vi "Process.vi"(8 "error in":errorcluster, 11 "MauiTemplate":refnum<class "MauiTemplate.lvclass">) -> (0 "error out":errorcluster, 3 "MauiTemplate out":refnum<class "MauiTemplate.lvclass">)   [LabVIEW 2016, in "MauiTemplate.lvclass"]
doc: "---------------------------------------------------------------\nJKI State Machine Objects™\nhttp://jki.net/state-machine-objects/\nCopyright (C) 2005-2015, JKI <info@jki.net>\nALL RIGHTS RESERVED"
uses:
  MauiTemplate.lvclass
  C:/Program Files (x86)/National Instruments/LabVIEW 2016/vi.lib/JKI/JKI SMO/SMO/SMO.lvclass
  C:/Program Files (x86)/National Instruments/LabVIEW 2016/vi.lib/Levylab/MAUI/MAUI.lvclass
  C:/Program Files (x86)/National Instruments/LabVIEW 2016/vi.lib/JKI/JKI SMO/SMO.UI/SMO.UI.lvclass
  <vilib>/JKI/JKI SMO/SMO/Typedefs/Parent Call--Enum.ctl
  <vilib>/Levylab/MAUI/Typedefs/PanelData.ctl
  <vilib>/Levylab/MAUI/MAUI.lvclass
  <vilib>/JKI/JKI SMO/SMO/SMO.lvclass
  <vilib>/JKI/JKI SMO/SMO.UI/SMO.UI.lvclass
panel:
  out "Title":string
  in  "Right Ring":u16(ring)
  in  "Left Ring":u16(ring)
  # "For instructions on how to use the JKI State Machine Objects, examples and video tutorials, visit:\nhttp://jki.net/state-machine-objects/\n\nJKI State Machine Objects™\nhttp://jki.net/state-machine-objects/\nCopyright (C) 2005-2015, JKI <info@jki.net>\nALL RIGHTS RESERVED"
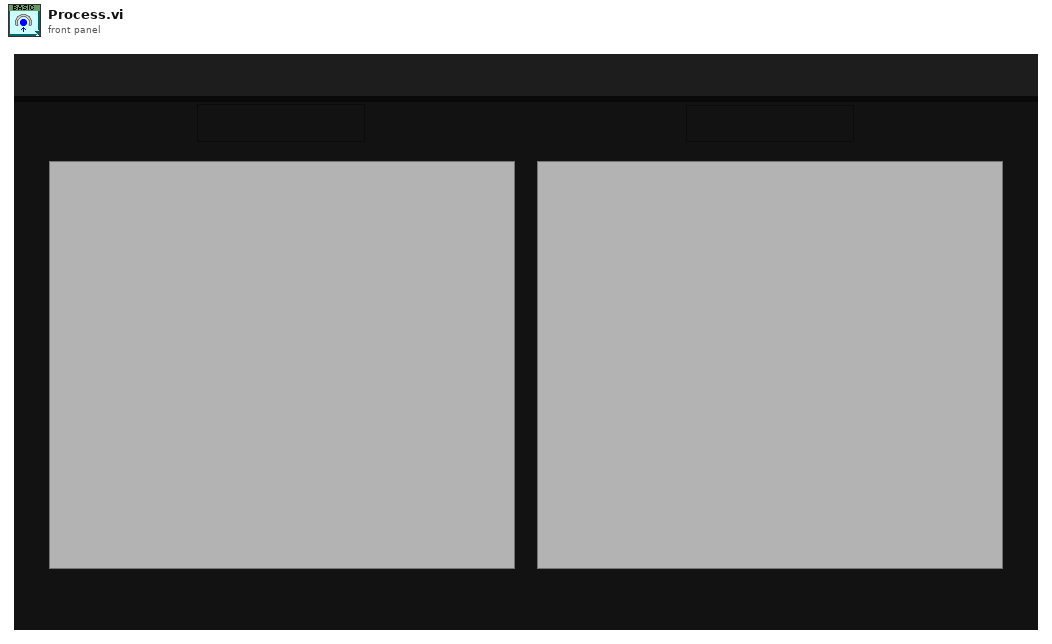
[diagram p1: front panel]
types:
  T1 = typedef "SMO.lvclass/Parent Call--Enum.ctl" = enum16{"Allows parent to run", "Does not request parent to run"}
  T2 = enum32{"invalid app kind", "Development System", "Run Time System", "Student Edition", "Embedded LabVIEW", "Evaluation", "Custom"}
  T3 = enum32{"Invalid", "Standard", "Closed", "Hidden", "Minimized", "Maximized"}
  T4 = enum32{"Bad", "Idle", "Run top level", "Running"}
  T5 = typedef "MAUI.lvclass/PanelData.ctl" = cluster{"Subpanel":refnum<vi>, "Ring":refnum<vi>, "Active":i32}
  T6 = cluster{"Core":cluster{"Current VI Reference":refnum<vi>, "Close Panel on Exit?":bool, "error":errorcluster}, "Self Reference":refnum<class "MauiTemplate.lvclass">, "Your string data":string, "Active Left":i32, "Active Right":i32}
  T7 = cluster{"Current VI Reference":refnum<vi>, "Close Panel on Exit?":bool, "error":errorcluster}
  T8 = typedef "SMO.lvclass/Protected Events.ctl" = cluster{"StopProcesses":refnum<user-event>, "AbortProcesses":refnum<user-event>, "Config Changed":refnum<user-event>, "Dependency":refnum<user-event>}
  T9 = typedef "MAUI.lvclass/PublicEvents--Cluster.ctl" = cluster{"ReadyForInfo ":refnum<user-event>}
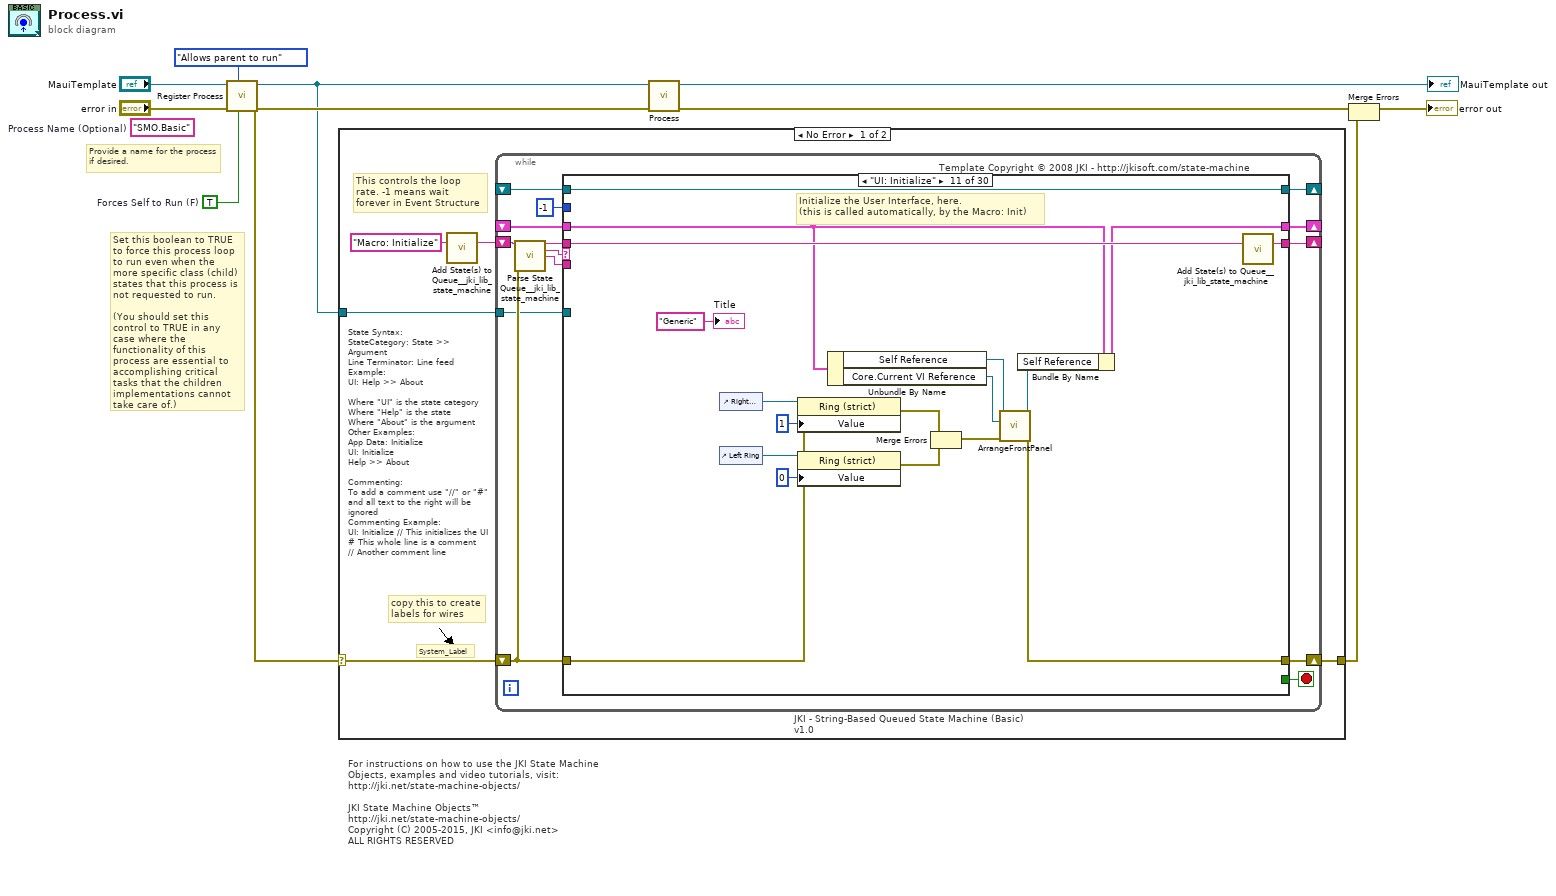
[diagram p0: block diagram]
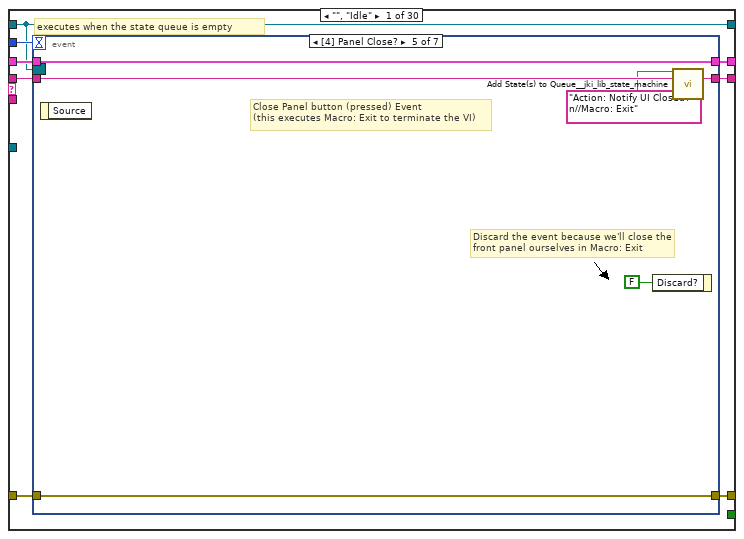
[diagram p2: hidden frame]
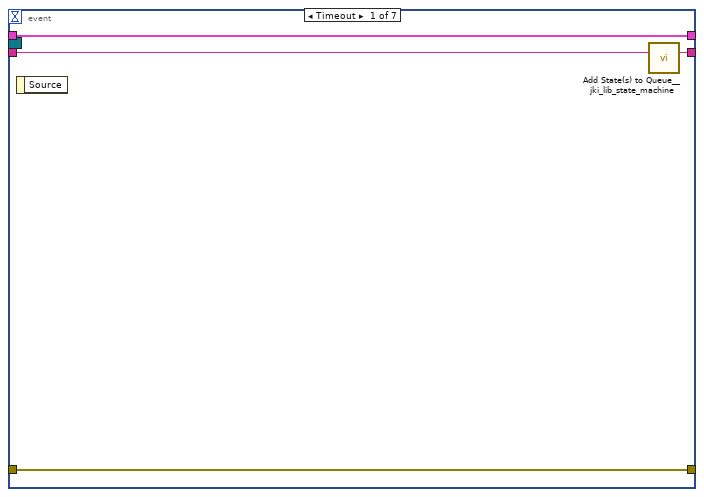
[diagram p3: hidden frame]
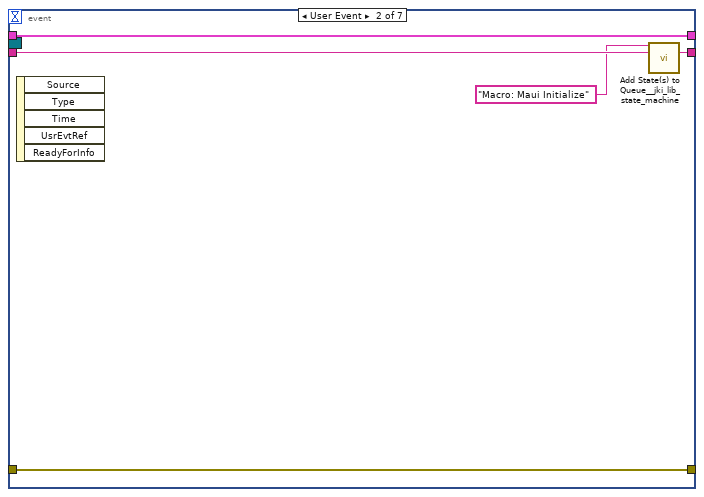
[diagram p4: hidden frame]
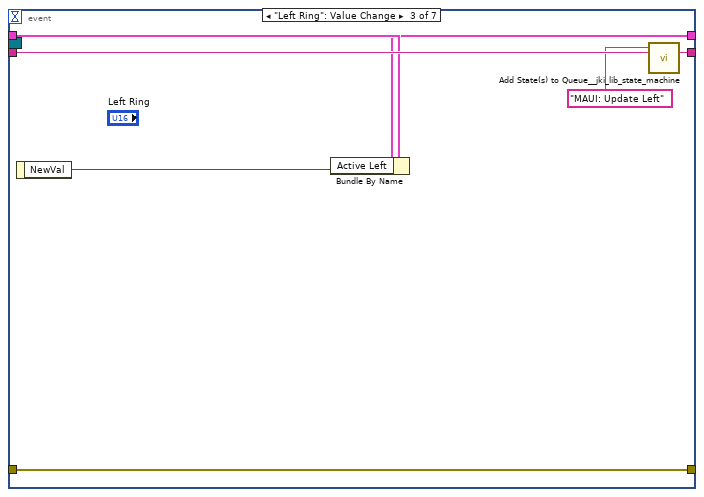
[diagram p5: hidden frame]
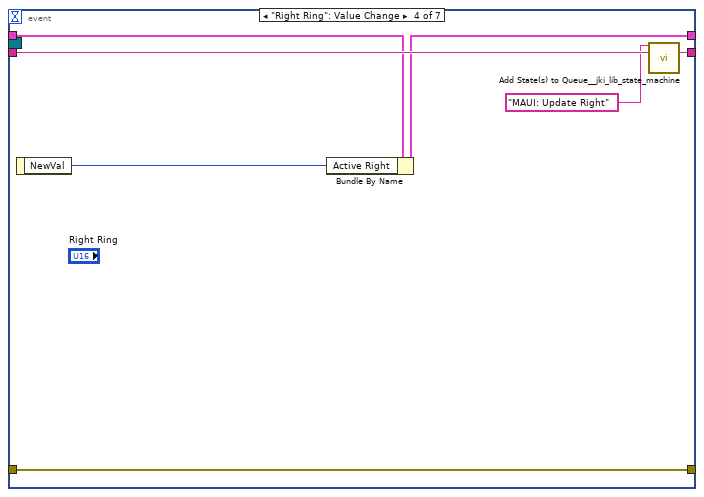
[diagram p6: hidden frame]
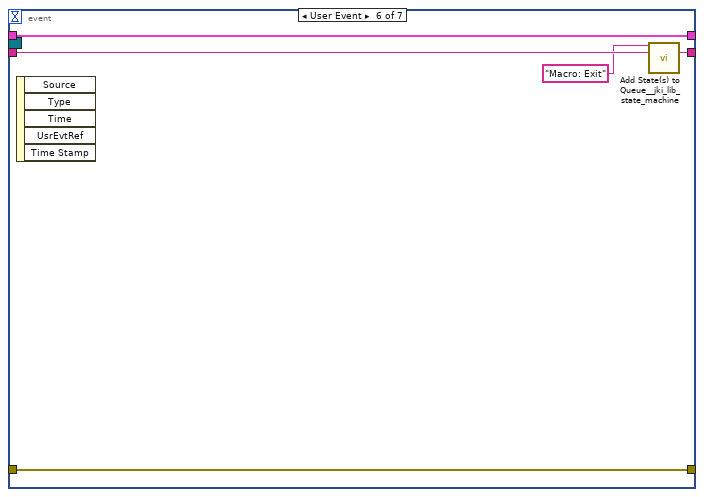
[diagram p7: hidden frame]
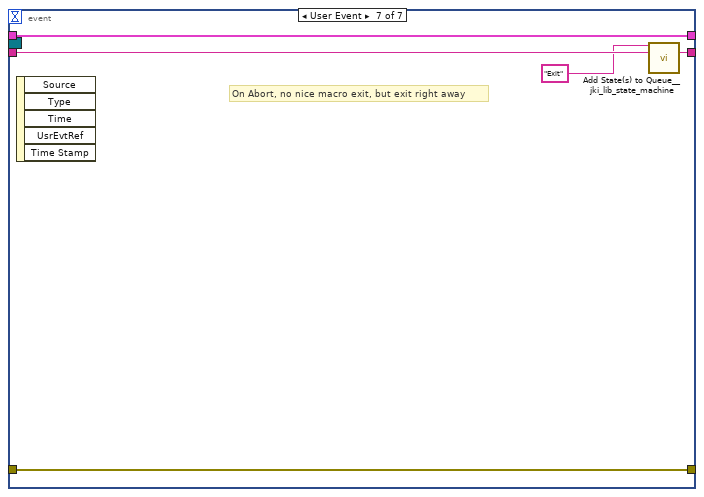
[diagram p8: hidden frame]
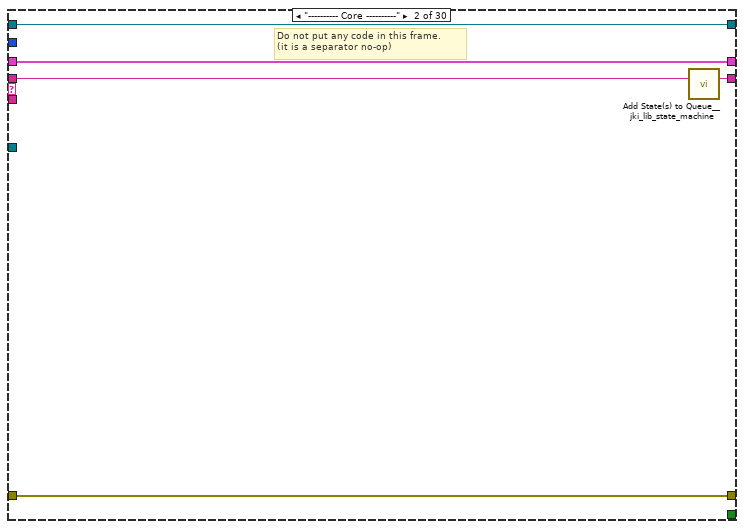
[diagram p9: hidden frame]
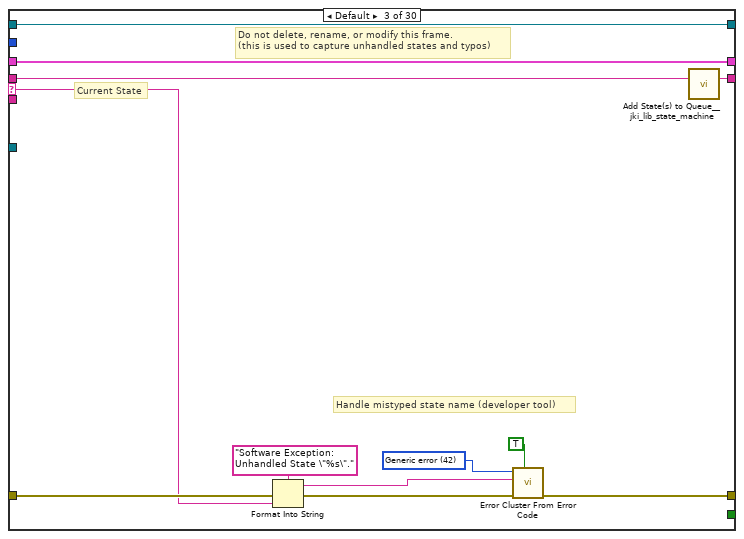
[diagram p10: hidden frame]
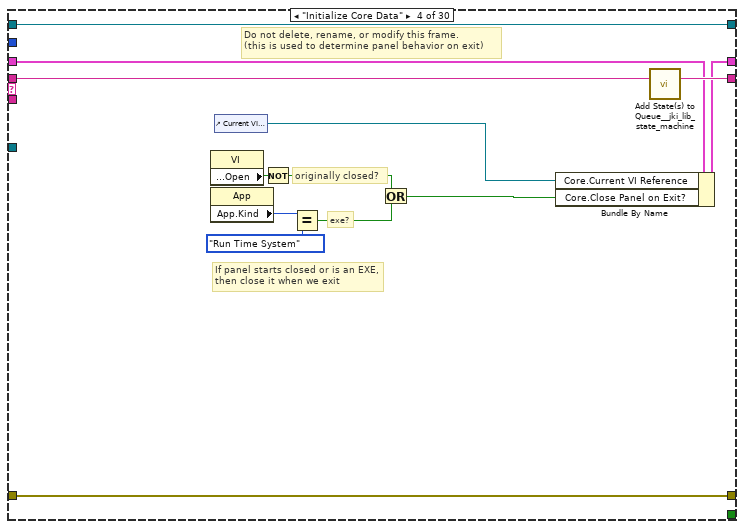
[diagram p11: hidden frame]
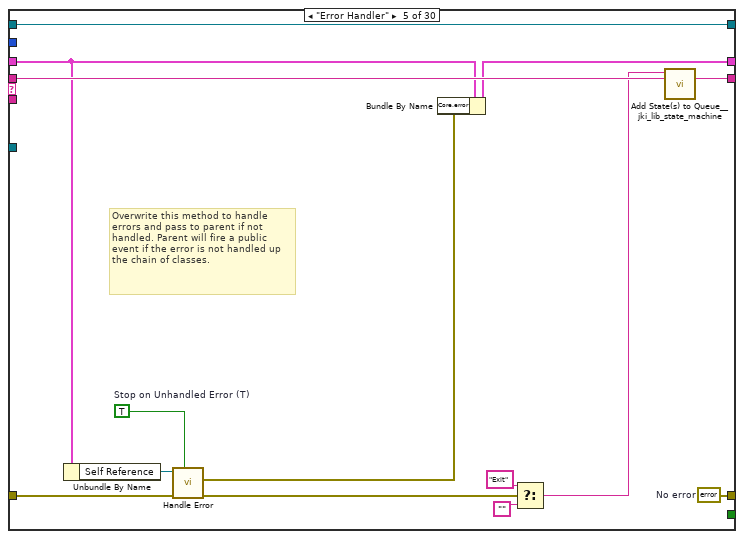
[diagram p12: hidden frame]
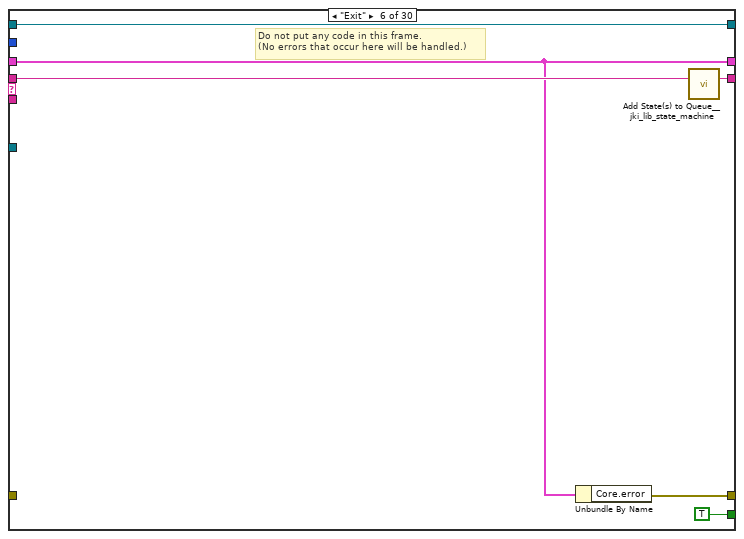
[diagram p13: hidden frame]
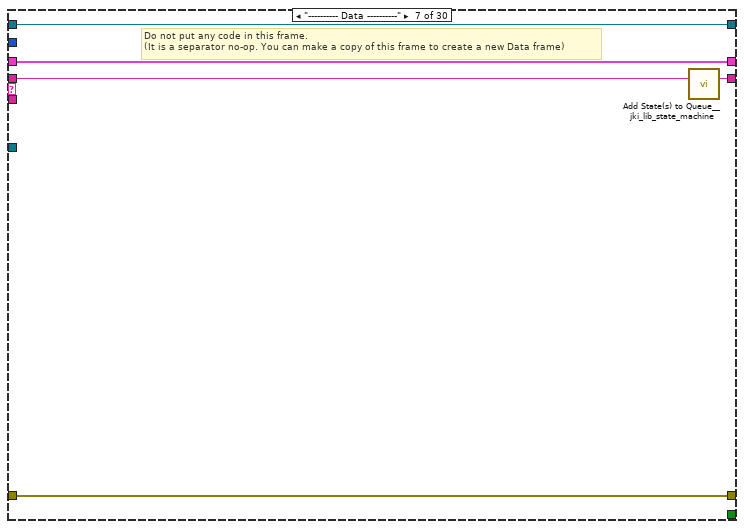
[diagram p14: hidden frame]
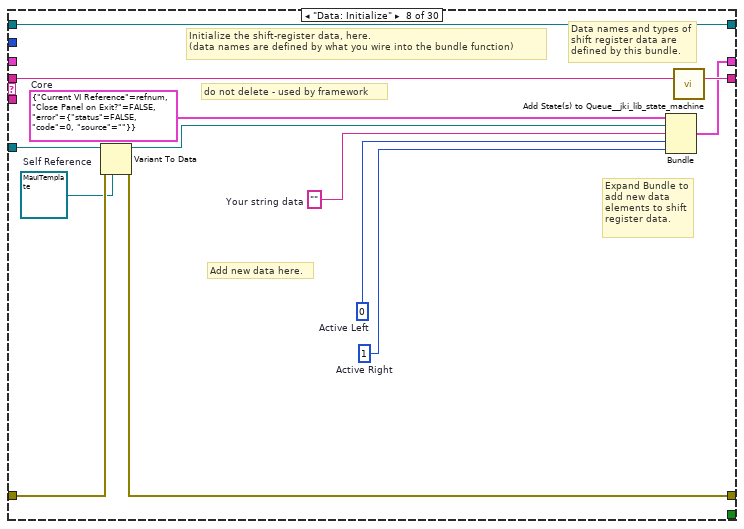
[diagram p15: hidden frame]
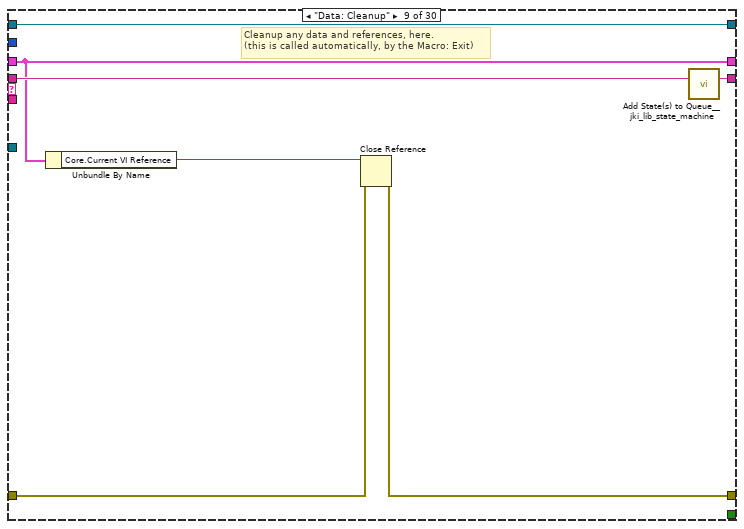
[diagram p16: hidden frame]
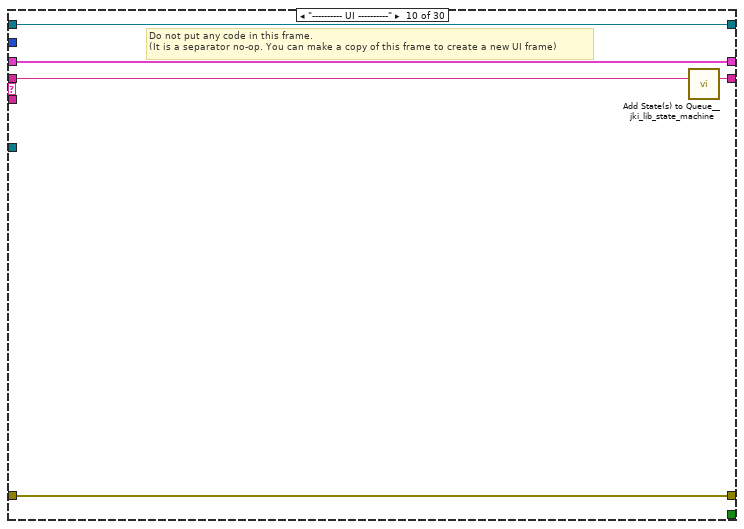
[diagram p17: hidden frame]
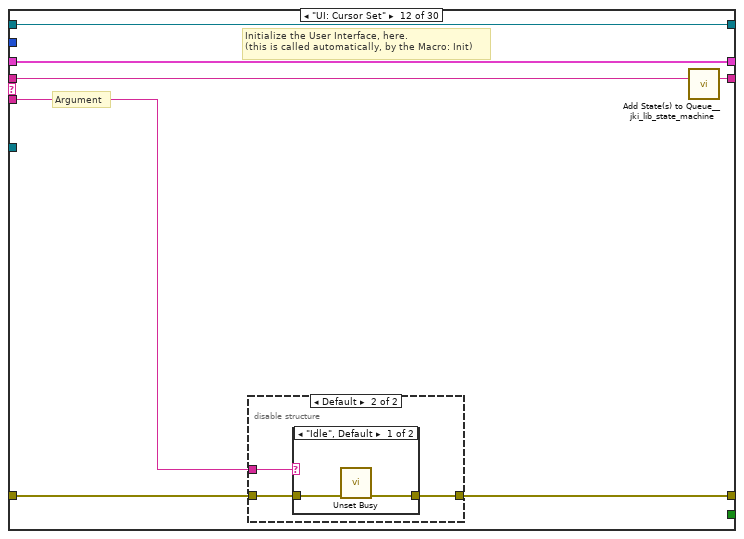
[diagram p18: hidden frame]
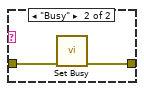
[diagram p20: hidden frame]
diagram:
  w2 = TRUE  # Forces Self to Run (F)
  (unwired) "SMO.Basic"  # Process Name (Optional)
  # "Provide a name for the process\nif desired."
  # "Set this boolean to TRUE to force this process loop to run even when the more specific class (child) states that this process is not requested to run.\n\n(You should set this control to TRUE in any case where the functionality of this process are essential to accomplishing critical tasks that the children implementations cannot take care of.)"
  # "For instructions on how to use the JKI State Machine Objects, examples and video tutorials, visit:\nhttp://jki.net/state-machine-objects/\n\nJKI State Machine Objects™\nhttp://jki.net/state-machine-objects/\nCopyright (C) 2005-2015, JKI <info@jki.net>\nALL RIGHTS RESERVED"
  n1 = call <vilib>:"Register Process.vi"("Forces Self to Run (F)"=w2, "Parent Call"=Parent_Call--Enum."Allows parent to run", "error in (no error)"="error in", "SMO"="MauiTemplate") -> ("error out"=w7:errorcluster, "SMO out"=w1:refnum<class "MauiTemplate.lvclass">)  [unwired: 6 in]
  n2 = case shown="No Error" w7 {
    selector: w7 -> [w12 w375]
    tunnel: w1 -> [w13 _]
    tunnel: [w11 w375] -> w4
    frame No Error {
      # "State Syntax:\nStateCategory: State >> Argument\nLine Terminator: Line feed\nExample:\nUI: Help >> About\n\nWhere \"UI\" is the state category\nWhere \"Help\" is the state\nWhere \"About\" is the argument\nOther Examples:\nApp Data: Initialize\nUI: Initialize\nHelp >> About\n\nCommenting:\nTo add a comment use \"//\" or \"#\" and all text to the right will be ignored\nCommenting Example:\nUI: Initialize // This initializes the UI\n# This whole line is a comment\n// Another comment line"
      # "copy this to create labels for wires"
      # "This controls the loop rate. -1 means wait forever in Event Structure"
      # "System_Label"
      n3 = call <vilib>:"Add State(s) to Queue__jki_lib_state_machine.vi"("State(s) in (\"\")"="Macro: Initialize") -> ("States Out"=w15:string)  [unwired: 14 in]
      n4 = while "JKI - String-Based Queued State Machine (Basic) v1.0" {
        shift-right: [w22] -> _
        shift-left: _ -> [w21]
        shift-right: [w25] -> w11
        shift-left: w12 -> [w19]
        shift-right: [w24] -> _
        shift-left: w15 -> [w26]
        tunnel: w13 -> [w18]
        shift-right: [w17] -> _
        shift-left: _ -> [w16]
        stop <- w23 stop-if-true
        # "Template Copyright © 2008 JKI - http://jkisoft.com/state-machine"
        n5 = call <vilib>:"Parse State Queue__jki_lib_state_machine.vi"("State Queue"=w26, "Error In (no error)"=w19) -> ("Remaining States"=w28:string, "Current State"=w29:string, "Arguments"=w27:string)  [unwired: 11 in]
        n6 = case shown="\"UI: Initialize\"" w29 {
          selector: w29 -> [_ _ w83 _ _ _ _ _ _ _ _ _ _ _ _ _ _ _ _ _ _ _ _ _ _ _ _ _ _ _]
          tunnel: w28 -> [w37 w81 w87 w106 w120 w126 w131 w144 w151 w156 w174 w181 w197 w229 w243 w249 w263 w268 w279 w284 w296 w302 w307 w314 w321 w326 w336 w346 w360 w374]
          tunnel: w27 -> [_ _ _ _ _ _ _ _ _ _ _ w175 w191 _ _ _ _ _ _ _ _ _ _ _ _ _ _ _ _ _]
          tunnel: w21 -> [w35 w78 w85 w97 w114 w122 w128 _ w146 w153 w168 w179 w193 w226 w239 w246 w254 w265 w276 w281 w294 w300 w305 w311 w317 w324 w333 w343 w352 w368]
          tunnel: [w34 w79 w89 w103 w115 w121 w129 w139 w147 w154 w164 w176 w194 w227 w241 w247 w261 w266 w270 w282 w290 w298 w303 w308 w318 w322 w328 w338 w354 w370] -> w25
          tunnel: w19 -> [w33 w79 w88 w103 w116 _ w129 w140 w148 w154 w160 w177 w195 w227 w241 w247 w261 w266 w271 w282 w291 w298 w303 w309 w318 w322 w327 w339 w355 w371]
          tunnel: [w36 w80 w86 w105 w119 w125 w130 w143 w150 w155 w173 w180 w196 w228 w242 w248 w262 w267 w278 w283 w295 w301 w306 w313 w320 w325 w335 w345 w359 w373] -> w24
          tunnel: [_ _ _ _ _ TRUE _ _ _ _ _ _ _ _ _ _ _ _ _ _ _ _ _ _ _ _ _ _ _ _] -> w23
          tunnel: [w32 w78 w85 w104 w113 w122 w128 w142 w146 w153 w167 w179 w193 w226 w239 w246 w254 w265 w276 w281 w294 w300 w305 w311 w316 w324 w332 w342 w351 w367] -> w22
          tunnel: -1 ("Timeout") -> [w31 _ _ _ _ _ _ _ _ _ _ _ _ _ _ _ _ _ _ _ _ _ _ _ _ _ _ _ _ _]
          tunnel: w18 -> [_ _ _ _ _ _ _ w137 _ _ _ _ _ _ _ _ _ _ _ _ _ _ _ _ _ _ _ _ _ _]
          tunnel: [w30 w77 w82 w94 w118 w123 w127 w135 w145 w152 w172 w178 w190 w225 w240 w245 w255 w264 w277 w280 w293 w299 w304 w312 w319 w323 w334 w344 w358 w372] -> w17
          tunnel: w16 -> [w30 w77 w82 w94 w118 w123 w127 w135 w145 w152 w172 w178 w190 w225 w240 w245 w255 w264 w277 w280 _ w299 w304 w312 w319 w323 w334 w344 w358 w372]
          frame "", "Idle" {
            # "executes when the state queue is empty"
            n7 = event shown="[4] Panel Close?" {
              selector: w30 -> [_ _ _ _ _ _ _]
              dyn-events: _ -> [_ _ _ _ _ _ _]
              timeout: w31 -> [_ _ _ _ _ _ _]
              tunnel: w37 -> [w41 w46 w53 w60 w66 w71 w76]
              tunnel: [w40 w45 w52 w59 w65 w70 w75] -> w36
              tunnel: w35 -> [w39 w44 w50 w57 w63 w68 w73]
              tunnel: [w38 w43 w51 w58 w64 w69 w74] -> w34
              tunnel: w33 -> [w38 w43 w51 w58 w64 w69 w74]
              tunnel: [w39 w44 w49 w56 w63 w68 w73] -> w32
              event Timeout {
                n8 = event-data() -> ()  [unwired: 1 in, 1 out]
                n9 = call <vilib>:"Add State(s) to Queue__jki_lib_state_machine.vi"("State(s) in (\"\")"=w41) -> ("States Out"=w40:string)  [unwired: 14 in]
              }
              event User Event {
                n10 = event-data() -> ()  [unwired: 1 in, 5 out]
                n11 = call <vilib>:"Add State(s) to Queue__jki_lib_state_machine.vi"("State(s) in Front (\"\")"="Macro: Maui Initialize", "State(s) in (\"\")"=w46) -> ("States Out"=w45:string)  [unwired: 13 in]
              }
              event "Left Ring": Value Change {
                n12 = event-data() -> ("NewVal"=w48:u16)  [unwired: 1 in]
                n13 = Bundle By Name(cluster=w50, "Active Left"=w48) -> (w49:T6)
                n14 = call <vilib>:"Add State(s) to Queue__jki_lib_state_machine.vi"("State(s) in Front (\"\")"="MAUI: Update Left", "State(s) in (\"\")"=w53) -> ("States Out"=w52:string)  [unwired: 13 in]
              }
              event "Right Ring": Value Change {
                n15 = event-data() -> ("NewVal"=w55:u16)  [unwired: 1 in]
                n16 = Bundle By Name(cluster=w57, "Active Right"=w55) -> (w56:T6)
                n17 = call <vilib>:"Add State(s) to Queue__jki_lib_state_machine.vi"("State(s) in Front (\"\")"="MAUI: Update Right", "State(s) in (\"\")"=w60) -> ("States Out"=w59:string)  [unwired: 13 in]
              }
              event Panel Close? {
                # "Discard the event because we'll close the front panel ourselves in Macro: Exit"
                # "Close Panel button (pressed) Event\n(this executes Macro: Exit to terminate the VI)"
                n18 = event-data() -> ()  [unwired: 1 in, 1 out]
                n19 = event-data("Discard?"=FALSE) -> ()  [unwired: 1 in, 1 out]
                n20 = call <vilib>:"Add State(s) to Queue__jki_lib_state_machine.vi"("State(s) in Front (\"\")"="Action: Notify UI Closed\n//Macro: Exit", "State(s) in (\"\")"=w66) -> ("States Out"=w65:string)  [unwired: 13 in]
              }
              event User Event {
                n21 = event-data() -> ()  [unwired: 1 in, 5 out]
                n22 = call <vilib>:"Add State(s) to Queue__jki_lib_state_machine.vi"("State(s) in Front (\"\")"="Macro: Exit", "State(s) in (\"\")"=w71) -> ("States Out"=w70:string)  [unwired: 13 in]
              }
              event User Event {
                # "On Abort, no nice macro exit, but exit right away"
                n23 = event-data() -> ()  [unwired: 1 in, 5 out]
                n24 = call <vilib>:"Add State(s) to Queue__jki_lib_state_machine.vi"("State(s) in Front (\"\")"="Exit", "State(s) in (\"\")"=w76) -> ("States Out"=w75:string)  [unwired: 13 in]
              }
            }
          }
          frame "---------- Core ----------" {
            # "Do not put any code in this frame.\n(it is a separator no-op)"
            n25 = call <vilib>:"Add State(s) to Queue__jki_lib_state_machine.vi"("State(s) in (\"\")"=w81) -> ("States Out"=w80:string)  [unwired: 14 in]
          }
          frame Default {
            w92 = 42 items=["No error", "Argument error", "Memory is full", "Out of zone", "End of file", "File already open", "Generic file I/O error", "File not found", "File permission error", "Disk is full", "Duplicate path", "Too many files open", "System feature not enabled", "Resource file not found", "Cannot add resource", "Resource not found", "Image not found", "Image memory error", "Pen does not exist", "Config type invalid", "Config token not found", "Config parse error", "Config memory error", "Bad external code format", "Bad external code offset", "External code not present", "Null window", "Destroy window error", "Null menu", "Print aborted", "Bad print record", "Print driver error", "Windows error during printing", "Memory error during printing", "Print dialog error", "Generic print error", "Invalid device refnum", "Device not found", "Device parameter error", "Device unit error", "Cannot open device", "Device call aborted", "Generic error", "Cancelled by user", "Object ID too low", "Object ID too high", "Object not in heap", "Unknown heap", "Unknown object (invalid DefProc)", "Unknown object (DefProc not in table)", "Message out of range", "Invalid (null) method", "Unknown message", "Manager call not supported", "Bad address", "Network operation in progress", "Network operation timed out", "Connection is busy", "Network attribute not supported", "Network error", "Address in use", "System out of memory", "Connection aborted", "Connection refused", "Not connected", "Already connected", "Connection closed", "Initialization error (interapplication manager)", "Bad occurrence", "Wait on unbound occurrence handler", "Occurrence queue overflow", "Datalog type conflict", "Unused", "Unrecognized type (interapplication manager)", "Memory corrupt", "Failed to make temporary DLL", "Old CIN version", "Drag socket not found", "Failed to load drop-object", "Failed to register OLE object", "Failed to release OLE object", "Format specifier type mismatch", "Unknown format specifier", "Too few format specifiers", "Too many format specifiers", "Scan failed", "Newer CIN version", "Error converting to variant", "Runtime menu error", "Password tampered", "Variant attribute not found", "Incompatible variant data type", "Event data is not available", "Event Store is not present", "Occurrence is not found", "Event Queue is not created", "Event info is not available", "Refnum passed is NULL", "Error retrieving Class GUID", "Error retrieving CoClass GUID", "Error retrieving TypeLib GUID.", "Bad built application magic bytes.", "Specific driver is different from the specific driver associated with the Logical Name.", "There is no session opened to the class driver.", "Max Error", "MAX - Error with config objects", "MAX - Error loading configuration", "MAX - Group not supported"]
            # "Current State"
            # "Do not delete, rename, or modify this frame.\n(this is used to capture unhandled states and typos)"
            # "Handle mistyped state name (developer tool)"
            n26 = Format Into String(format string="Software Exception: Unhandled State \"%s\"." ("message"), error in=w88, w83) -> (resulting string=w91:string, error out=w90:errorcluster)  [unwired: 1 in]
            n27 = call <vilib>:"Error Cluster From Error Code.vi"("show call chain? (False)"=TRUE, "error in (no error)"=w90, "error message (\"\")"=w91, "error code (0)"=w92) -> ("error out"=w89:errorcluster)  [unwired: 5 in]
            n28 = call <vilib>:"Add State(s) to Queue__jki_lib_state_machine.vi"("State(s) in (\"\")"=w87) -> ("States Out"=w86:string)  [unwired: 14 in]
          }
          frame "Initialize Core Data" {
            # "Do not delete, rename, or modify this frame.\n(this is used to determine panel behavior on exit)"
            # "originally closed?"
            # "exe?"
            # "If panel starts closed or is an EXE, then close it when we exit"
            n29 = property class="VI"() -> ("Front Panel.Open"=w102:bool)  [unwired: 2 in, 2 out]
            n30 = property class="App"() -> ("App.Kind"=w101:T2)  [unwired: 2 in, 2 out]
            n31 = control-ref of="Current VI Reference"() -> (w95:refnum<vi>)
            n32 = Not(x=w102) -> (.not. x?=w99:bool)
            n33 = Equal?(x=w101, y=T2."Run Time System" ("Application:Kind")) -> (x = y?=w98:bool)
            n34 = Or(x=w99, y=w98) -> (x .or. y?=w96:bool)
            n35 = Bundle By Name(cluster=w97, "Core.Current VI Reference"=w95, "Core.Close Panel on Exit?"=w96) -> (w104:T6)
            n36 = call <vilib>:"Add State(s) to Queue__jki_lib_state_machine.vi"("State(s) in (\"\")"=w106) -> ("States Out"=w105:string)  [unwired: 14 in]
          }
          frame "Error Handler" {
            w107 = TRUE  # Stop on Unhandled Error (T)
            w115 = errorcluster {"status"=FALSE, "code"=0, "source"=""}  # No error
            # "Overwrite this method to handle errors and pass to parent if not handled. Parent will fire a public event if the error is not handled up the chain of classes."
            n37 = Unbundle By Name(w114) -> ("Self Reference"=w117:refnum<class "MauiTemplate.lvclass">)
            n38 = call-dynamic "Handle Error.vi"("Stop on Unhandled Error (T)"=w107, "error in"=w116, "SMO"=w117) -> ("handling error"=w108:errorcluster, "Unhandled error"=w111:errorcluster)  [unwired: 6 in, 1 out]
            n39 = Bundle By Name(cluster=w114, "Core.error"=w111) -> (w113:T6)
            n40 = Select(t="Exit", s=w108, f="") -> (s? t:f=w112:string)
            n41 = call <vilib>:"Add State(s) to Queue__jki_lib_state_machine.vi"("State(s) in Front (\"\")"=w112, "State(s) in (\"\")"=w120) -> ("States Out"=w119:string)  [unwired: 13 in]
          }
          frame "Exit" {
            # "Do not put any code in this frame.\n(No errors that occur here will be handled.)"
            n42 = Unbundle By Name(w122) -> ("Core.error"=w121:errorcluster)
            n43 = call <vilib>:"Add State(s) to Queue__jki_lib_state_machine.vi"("State(s) in (\"\")"=w126) -> ("States Out"=w125:string)  [unwired: 14 in]
          }
          frame "---------- Data ----------" {
            # "Do not put any code in this frame.\n(It is a separator no-op. You can make a copy of this frame to create a new Data frame)"
            n44 = call <vilib>:"Add State(s) to Queue__jki_lib_state_machine.vi"("State(s) in (\"\")"=w131) -> ("States Out"=w130:string)  [unwired: 14 in]
          }
          frame "Data: Initialize" {
            w132 = 1  # Active Right
            w133 = 0  # Active Left
            w134 = T7 {"Current VI Reference"=refnum, "Close Panel on Exit?"=FALSE, "error"={"status"=FALSE, "code"=0, "source"=""}}  # Core
            w138 = refnum<class "MauiTemplate.lvclass"> refnum  # Self Reference
            w141 = ""  # Your string data
            # "do not delete - used by framework"
            # "Expand Bundle to add new data elements to shift register data."
            # "Add new data here."
            # "Data names and types of shift register data are defined by this bundle."
            # "Initialize the shift-register data, here.\n(data names are defined by what you wire into the bundle function)"
            n45 = Variant To Data(error in=w140, type=w138, Variant=w137) -> (data=w136:refnum<class "MauiTemplate.lvclass">, error out=w139:errorcluster)
            n46 = Bundle("Core"=w134, "Self Reference"=w136, "Your string data"=w141, "Active Left"=w133, "Active Right"=w132) -> (w142:T6)  [unwired: 1 in]
            n47 = call <vilib>:"Add State(s) to Queue__jki_lib_state_machine.vi"("State(s) in (\"\")"=w144) -> ("States Out"=w143:string)  [unwired: 14 in]
          }
          frame "Data: Cleanup" {
            # "Cleanup any data and references, here.\n(this is called automatically, by the Macro: Exit)"
            n48 = Unbundle By Name(w146) -> ("Core.Current VI Reference"=w149:refnum<vi>)
            n49 = Close Reference(reference=w149, error in (no error)=w148) -> (error out=w147:errorcluster)
            n50 = call <vilib>:"Add State(s) to Queue__jki_lib_state_machine.vi"("State(s) in (\"\")"=w151) -> ("States Out"=w150:string)  [unwired: 14 in]
          }
          frame "---------- UI ----------" {
            # "Do not put any code in this frame.\n(It is a separator no-op. You can make a copy of this frame to create a new UI frame)"
            n51 = call <vilib>:"Add State(s) to Queue__jki_lib_state_machine.vi"("State(s) in (\"\")"=w156) -> ("States Out"=w155:string)  [unwired: 14 in]
          }
          frame "UI: Initialize" {
            # "Initialize the User Interface, here.\n(this is called automatically, by the Macro: Init)"
            n52 = control-ref of="Right Ring"() -> (w171:refnum<vi>)
            n53 = control-ref of="Left Ring"() -> (w162:refnum<vi>)
            n54 = property class="Ring (strict)"(reference=w171, error in=w160, "Value"=u16 1) -> (error out=w157:errorcluster)  [unwired: 1 out]
            n55 = property class="Ring (strict)"(reference=w162, error in=w160, "Value"=u16 0) -> (error out=w158:errorcluster)  [unwired: 1 out]
            n56 = Unbundle By Name(w168) -> ("Self Reference"=w169:refnum<class "MauiTemplate.lvclass">, "Core.Current VI Reference"=w165:refnum<vi>)
            n57 = Merge Errors(w157, w158) -> (w159:errorcluster)
            n58 = call <vilib>:"ArrangeFrontPanel.vi"("error in (no error)"=w159, "This VI"=w165, "MAUI in"=w169) -> ("error out"=w164:errorcluster, "MAUI out"=w166:refnum<class "MauiTemplate.lvclass">)  [unwired: 7 in]
            n59 = Bundle By Name(cluster=w168, "Self Reference"=w166) -> (w167:T6)
            n60 = call <vilib>:"Add State(s) to Queue__jki_lib_state_machine.vi"("State(s) in (\"\")"=w174) -> ("States Out"=w173:string)  [unwired: 14 in]
            "Title" <- "Generic" ("Title")
          }
          frame "UI: Cursor Set" {
            # "Argument"
            # "Initialize the User Interface, here.\n(this is called automatically, by the Macro: Init)"
            n61 = disable-structure shown="Default" {
              disable-tunnel: w177 -> [w182 w185]
              disable-tunnel: [w182 w184] -> w176
              disable-tunnel: w175 -> [_ w183]
              frame condition #0 {
              }
              frame condition #1 (active) {
                n62 = case shown="\"Idle\", Default" w183 {
                  tunnel: w185 -> [w187 w189]
                  tunnel: [w186 w188] -> w184
                  frame "Idle", Default {
                    n63 = call <vilib>:"Unset Busy.vi"("error in (no error)"=w187) -> ("error out"=w186:errorcluster)  [unwired: 10 in]
                  }
                  frame "Busy" {
                    n64 = call <vilib>:"Set Busy.vi"("error in (no error)"=w189) -> ("error out"=w188:errorcluster)  [unwired: 9 in, 1 out]
                  }
                }
              }
            }
            n65 = call <vilib>:"Add State(s) to Queue__jki_lib_state_machine.vi"("State(s) in (\"\")"=w181) -> ("States Out"=w180:string)  [unwired: 14 in]
          }
          frame "UI: Front Panel State" {
            # "Argument"
            # "Set Front Panel Open or Closed\n(Usage: \"UI: Front Panel State >> Open|Close\")"
            n66 = Unbundle By Name(w193) -> ("Core.Current VI Reference"=w192:refnum<vi>)
            n67 = disable-structure shown="Default" {
              disable-tunnel: w195 -> [w201 w224]
              disable-tunnel: [w200 w224] -> w194
              disable-tunnel: w192 -> [w199 _]
              disable-tunnel: w191 -> [w198 _]
              frame condition #0 (active) {
                n68 = case shown="\"Close\"" w198 {
                  tunnel: w201 -> [w205 w218]
                  tunnel: [w207 w219] -> w200
                  tunnel: w199 -> [w206 w216]
                  frame "Open", Default {
                    n69 = property class="VI"(reference=w206, error in=w205) -> (reference out=w203:refnum<vi>, error out=w204:errorcluster, "FP.State"=w202:T3)
                    n70 = case shown="\"Closed\"" w202 {
                      tunnel: [w210 w213] -> w207
                      tunnel: w204 -> [w209 w213]
                      tunnel: w203 -> [w208 _]
                      frame "Closed" {
                        n71 = invoke class="VI" method="FP.Open"(reference=w208, error in=w209, "Activate"=TRUE, "State"=T3."Standard") -> (error out=w210:errorcluster)  [unwired: 1 in, 4 out]
                      }
                      frame Default {
                      }
                    }
                  }
                  frame "Close" {
                    n72 = property class="VI"(reference=w216, error in=w218) -> (reference out=w215:refnum<vi>, error out=w217:errorcluster, "FP.State"=w214:T3)
                    n73 = case shown="Default" w214 {
                      tunnel: [w220 w223] -> w219
                      tunnel: w217 -> [w220 w222]
                      tunnel: w215 -> [_ w221]
                      frame "Invalid", "Closed" {
                      }
                      frame Default {
                        n74 = invoke class="VI" method="FP.Close"(reference=w221, error in=w222) -> (error out=w223:errorcluster)  [unwired: 1 in, 2 out]
                      }
                    }
                  }
                }
              }
              frame condition #1 {
              }
            }
            n75 = call <vilib>:"Add State(s) to Queue__jki_lib_state_machine.vi"("State(s) in (\"\")"=w197) -> ("States Out"=w196:string)  [unwired: 14 in]
          }
          frame "---------- Macro ----------" {
            # "Do not put any code in this frame.\n(It is a separator no-op. You can make a copy of this frame to create a new Macro frame)"
            n76 = call <vilib>:"Add State(s) to Queue__jki_lib_state_machine.vi"("State(s) in (\"\")"=w229) -> ("States Out"=w228:string)  [unwired: 14 in]
          }
          frame "Macro: Initialize" {
            w234 = "UI: Initialize\nUI: Front Panel State >> Open"  # UI: Initialize UI: Front Panel State >> Open
            w230 = "Process: Sync"
            # "Initialization Macro\n(This is called once, when the VI starts)"
            n77 = control-ref of="This VI"() -> (w232:refnum<vi>)
            n78 = property class="VI"(reference=w232) -> ("Exec.State"=w231:T4)  [unwired: 1 in, 2 out]
            n79 = Equal?(x=w231, y=T4."Run top level") -> (x = y?=w237:bool)
            n80 = Select(t=w230, s=w237, f="") -> ()  [unwired: 1 out]
            n81 = call <vilib>:"Add State(s) to Queue__jki_lib_state_machine.vi"("State(s) in Front (\"\")"="Data: Initialize\nInitialize Core Data\nEvents: Register", "State(s) in (\"\")"=w230, "State(s) at Back (\"\")"=w234) -> ("States Out"=w233:string)  [unwired: 12 in]
            n82 = call <vilib>:"Add State(s) to Queue__jki_lib_state_machine.vi"("State(s) in Front (\"\")"=w233, "State(s) in (\"\")"=w243) -> ("States Out"=w242:string)  [unwired: 13 in]
          }
          frame "Macro: Maui Initialize" {
            # "Do not put any code in this frame.\n(It is a separator no-op. You can make a copy of this frame to create a new Macro frame)"
            n83 = call <vilib>:"Add State(s) to Queue__jki_lib_state_machine.vi"("State(s) in Front (\"\")"="MAUI: Send Left\nMAUI: Send Right\nMAUI: Update Left\nMAUI: Update Right", "State(s) in (\"\")"=w249) -> ("States Out"=w248:string)  [unwired: 13 in]
          }
          frame "Macro: Exit" {
            # "Exit Macro\n(This is called once, when the VI exits)"
            n84 = Unbundle By Name(w254) -> ("Core.Close Panel on Exit?"=w260:bool)
            n85 = Select(t="UI: Front Panel State >> Close", s=w260, f="") -> (s? t:f=w257:string)
            n86 = call <vilib>:"Add State(s) to Queue__jki_lib_state_machine.vi"("State(s) in Front (\"\")"="Data: Cleanup\nEvents: Unregister", "State(s) in (\"\")"="Process: Sync", "State(s) at Back (\"\")"="Exit") -> ("States Out"=w251:string)  [unwired: 12 in]
            n87 = call <vilib>:"Add State(s) to Queue__jki_lib_state_machine.vi"("State(s) in (\"\")"=w257, "State(s) at Back (\"\")"=w251) -> ("States Out"=w256:string)  [unwired: 13 in]
            n88 = call <vilib>:"Add State(s) to Queue__jki_lib_state_machine.vi"("State(s) in Front (\"\")"=w256, "State(s) in (\"\")"=w263) -> ("States Out"=w262:string)  [unwired: 13 in]
          }
          frame "---------- Process ----------" {
            # "Template Separator\n(You can make a copy of, or modify, this frame)"
            n89 = call <vilib>:"Add State(s) to Queue__jki_lib_state_machine.vi"("State(s) in (\"\")"=w268) -> ("States Out"=w267:string)  [unwired: 14 in]
          }
          frame "Process: Sync" {
            n90 = Unbundle By Name(w276) -> ("Self Reference"=w272:refnum<class "MauiTemplate.lvclass">)
            n91 = call <vilib>:"WaitOnProcessSync.vi"("error in (no error)"=w271, "SMO"=w272) -> ("error out"=w270:errorcluster, "Don't run?"=w275:bool)  [unwired: 7 in, 1 out]
            n92 = Select(t="Data: Cleanup\nEvents: Unregister\nExit", s=w275, f="") -> (s? t:f=w269:string)
            n93 = call <vilib>:"Add State(s) to Queue__jki_lib_state_machine.vi"("State(s) in Front (\"\")"=w269, "State(s) in (\"\")"=w279) -> ("States Out"=w278:string)  [unwired: 13 in]
          }
          frame "---------- Events ----------" {
            # "Template Separator\n(You can make a copy of, or modify, this frame)"
            n94 = call <vilib>:"Add State(s) to Queue__jki_lib_state_machine.vi"("State(s) in (\"\")"=w284) -> ("States Out"=w283:string)  [unwired: 14 in]
          }
          frame "Events: Register" {
            # "Expand to add\nmore events"
            n95 = Unbundle By Name(w294) -> ("Self Reference"=w287:refnum<class "MauiTemplate.lvclass">)
            n96 = call <vilib>:"GetProtectedEvents.vi"("SMO"=w287) -> ("error out"=w288:errorcluster, "SMO Protected Events"=w292:T8)  [unwired: 8 in, 1 out]
            n97 = call <vilib>:"MAUI.GetPublicEvents.vi"("MAUI"=w287) -> ("error out"=w285:errorcluster, "Public Events"=w286:T9)  [unwired: 8 in, 1 out]
            n98 = register-events(w292, w286) -> (reference out=w293:refnum<event-registration>, error out=w289:errorcluster)  [unwired: 2 in]
            n99 = Merge Errors(w291, w289, w288, w285) -> (w290:errorcluster)
            n100 = call <vilib>:"Add State(s) to Queue__jki_lib_state_machine.vi"("State(s) in (\"\")"=w296) -> ("States Out"=w295:string)  [unwired: 14 in]
          }
          frame "Events: Unregister" {
            n101 = Unregister For Events(event registration refnum=w299, error in=w298) -> (error out=w297:errorcluster)
            n102 = call <vilib>:"Clear Errors.vi"("error in (no error)"=w297) -> ()  [unwired: 5 in, 2 out]
            n103 = call <vilib>:"Add State(s) to Queue__jki_lib_state_machine.vi"("State(s) in (\"\")"=w302) -> ("States Out"=w301:string)  [unwired: 14 in]
          }
          frame "---------- Action ----------" {
            n104 = call <vilib>:"Add State(s) to Queue__jki_lib_state_machine.vi"("State(s) in (\"\")"=w307) -> ("States Out"=w306:string)  [unwired: 14 in]
          }
          frame "Action: Notify UI Closed" {
            n105 = Unbundle By Name(w311) -> ("Self Reference"=w310:refnum<class "MauiTemplate.lvclass">)
            n106 = call <vilib>:"Hide.vi"("error in (no error)"=w309, "SMO.UI"=w310) -> ("error out"=w308:errorcluster)  [unwired: 8 in, 1 out]
            n107 = call <vilib>:"Add State(s) to Queue__jki_lib_state_machine.vi"("State(s) in (\"\")"=w314) -> ("States Out"=w313:string)  [unwired: 14 in]
          }
          frame "Action: Template" {
            n108 = Unbundle By Name(w317) -> ("Self Reference"=w315:refnum<class "MauiTemplate.lvclass">)
            n109 = Bundle By Name(cluster=w317, "Self Reference"=w315) -> (w316:T6)
            n110 = call <vilib>:"Add State(s) to Queue__jki_lib_state_machine.vi"("State(s) in (\"\")"=w321) -> ("States Out"=w320:string)  [unwired: 14 in]
          }
          frame "---------- MAUI ----------" {
            n111 = call <vilib>:"Add State(s) to Queue__jki_lib_state_machine.vi"("State(s) in (\"\")"=w326) -> ("States Out"=w325:string)  [unwired: 14 in]
          }
          frame "MAUI: Update Left" {
            n112 = Unbundle By Name(w333) -> ("Self Reference"=w331:refnum<class "MauiTemplate.lvclass">, "Active Left"=w329:i32)
            n113 = call <vilib>:"MAUI.UpdateLeftSubpanel.vi"("error in (no error)"=w327, "Update Left Subpanel"=w329, "MAUI"=w331) -> ("error out"=w328:errorcluster, "MAUI out"=w330:refnum<class "MauiTemplate.lvclass">)  [unwired: 7 in]
            n114 = Bundle By Name(cluster=w333, "Self Reference"=w330) -> (w332:T6)
            n115 = call <vilib>:"Add State(s) to Queue__jki_lib_state_machine.vi"("State(s) in (\"\")"=w336) -> ("States Out"=w335:string)  [unwired: 14 in]
          }
          frame "MAUI: Update Right" {
            n116 = Unbundle By Name(w343) -> ("Self Reference"=w340:refnum<class "MauiTemplate.lvclass">, "Active Right"=w337:i32)
            n117 = call <vilib>:"MAUI.UpdateRightSubpanel.vi"("error in (no error)"=w339, "UpdateRightSubpanel"=w337, "MAUI"=w340) -> ("error out"=w338:errorcluster, "MAUI out"=w341:refnum<class "MauiTemplate.lvclass">)  [unwired: 7 in]
            n118 = Bundle By Name(cluster=w343, "Self Reference"=w341) -> (w342:T6)
            n119 = call <vilib>:"Add State(s) to Queue__jki_lib_state_machine.vi"("State(s) in (\"\")"=w346) -> ("States Out"=w345:string)  [unwired: 14 in]
          }
          frame "MAUI: Send Left" {
            w356 = 0  # Active
            n120 = control-ref of="Left Subpanel"() -> (w348:refnum<vi>)
            n121 = control-ref of="Left Ring"() -> (w349:refnum<vi>)
            n122 = Unbundle By Name(w352) -> ("Self Reference"=w353:refnum<class "MauiTemplate.lvclass">)
            n123 = Bundle(cluster=T5 {"Subpanel"=refnum, "Ring"=refnum, "Active"=0} ("Panel"), "Subpanel"=w348, "Ring"=w349, "Active"=w356) -> (w357:T5)
            n124 = call <vilib>:"WriteLeftData.vi"("error in (no error)"=w355, "Left"=w357, "MAUI in"=w353) -> ("error out"=w354:errorcluster, "MAUI out"=w350:refnum<class "MauiTemplate.lvclass">)  [unwired: 7 in]
            n125 = Bundle By Name(cluster=w352, "Self Reference"=w350) -> (w351:T6)
            n126 = call <vilib>:"Add State(s) to Queue__jki_lib_state_machine.vi"("State(s) in (\"\")"=w360) -> ("States Out"=w359:string)  [unwired: 14 in]
          }
          frame "MAUI: Send Right" {
            n127 = Unbundle By Name(w368) -> ("Self Reference"=w369:refnum<class "MauiTemplate.lvclass">)
            n128 = control-ref of="Right Subpanel"() -> (w362:refnum<vi>)
            n129 = control-ref of="Right Ring"() -> (w363:refnum<vi>)
            n130 = Bundle(cluster=T5 {"Subpanel"=refnum, "Ring"=refnum, "Active"=0} ("Panel"), "Subpanel"=w362, "Ring"=w363, "Active"=1) -> (w361:T5)
            n131 = call <vilib>:"WriteRightData.vi"("error in (no error)"=w371, "Panel"=w361, "MAUI in"=w369) -> ("error out"=w370:errorcluster, "MAUI out"=w366:refnum<class "MauiTemplate.lvclass">)  [unwired: 7 in]
            n132 = Bundle By Name(cluster=w368, "Self Reference"=w366) -> (w367:T6)
            n133 = call <vilib>:"Add State(s) to Queue__jki_lib_state_machine.vi"("State(s) in (\"\")"=w374) -> ("States Out"=w373:string)  [unwired: 14 in]
          }
        }
      }
    }
    frame Error {
    }
  }
  n134 = call-parent "Process.vi"("error in"=w7, "MAUI"=w1) -> ("error out"=w5:errorcluster, "MAUI out"=→"MauiTemplate out":refnum<class "MauiTemplate.lvclass">)  [unwired: 8 in]
  n135 = Merge Errors(w5, w4) -> (→"error out":errorcluster)
